vi "Build Update Query.vi"(6 "Where":string, 7 "Schema Name":string, 8 "error in (no error)":errorcluster, 9 "Data":string[](array[string]), 10 "Column Names":string[](array[string]), 11 "Table Name":string) -> (0 "error out":errorcluster, 3 "SQL":string caption="SQL+ (Col[]) VALUES (?[])")   [LabVIEW 2023, in "HardwareAbstractionLayer_LVOOP.lvlib" / "Database.lvclass"]
uses:
  Database.lvclass
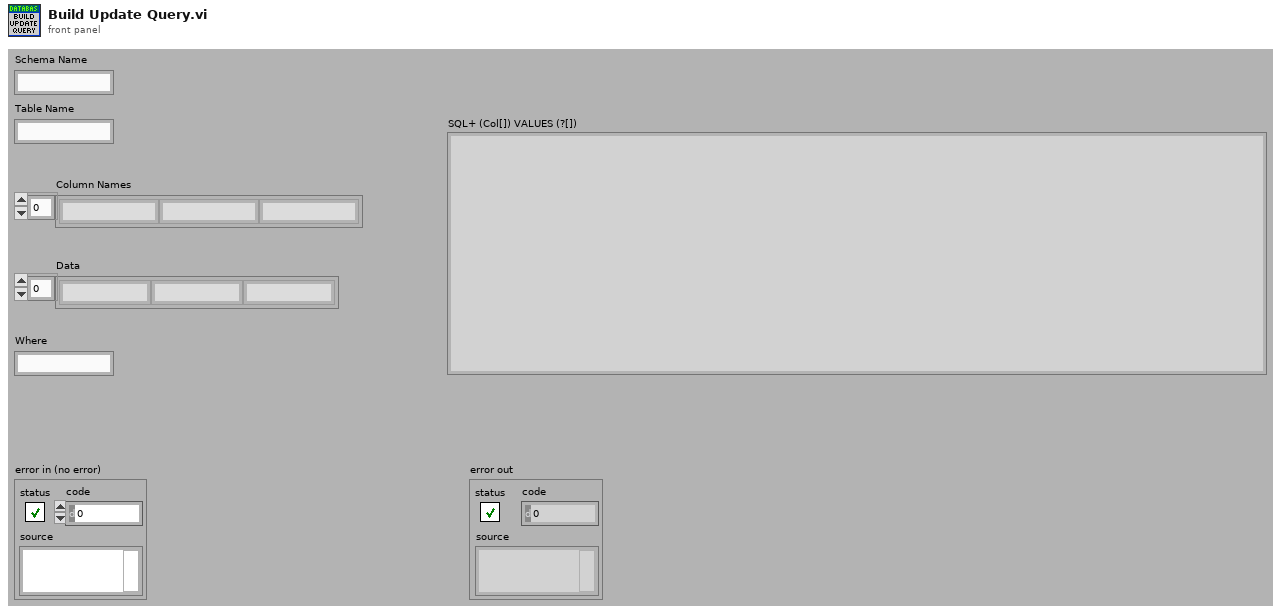
[diagram p1: front panel]
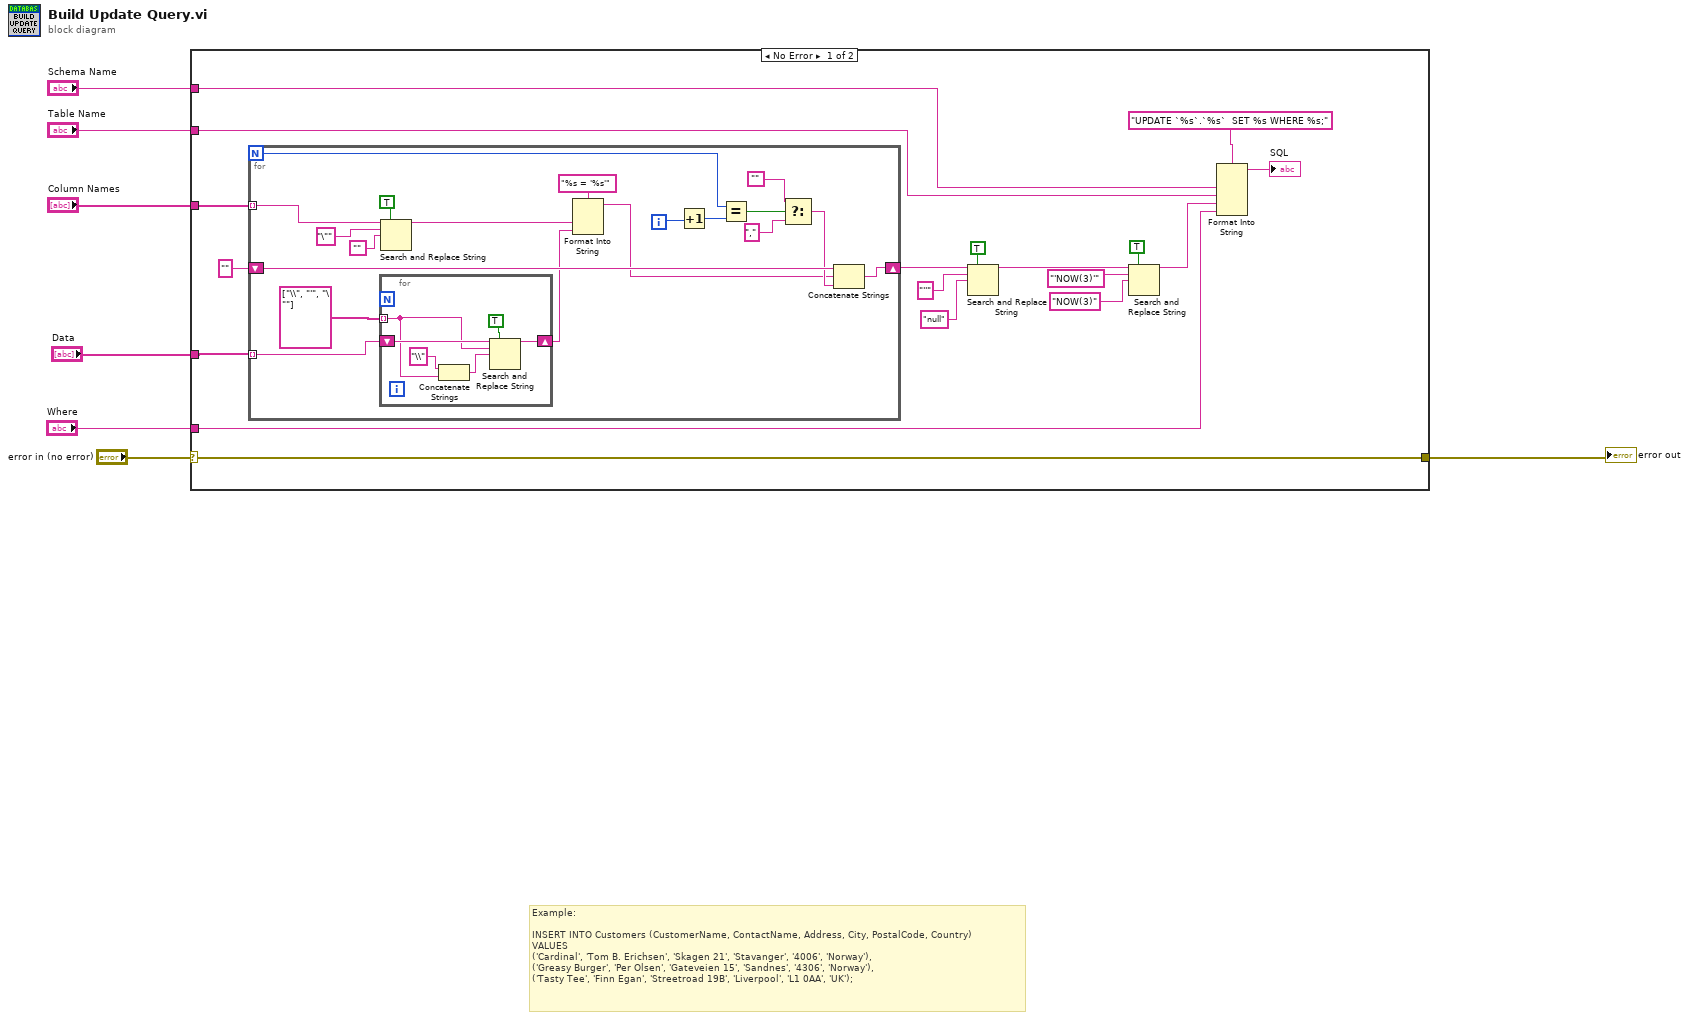
[diagram p0: block diagram]
diagram:
  # "Example:\n\nINSERT INTO Customers (CustomerName, ContactName, Address, City, PostalCode, Country)\nVALUES\n('Cardinal', 'Tom B. Erichsen', 'Skagen 21', 'Stavanger', '4006', 'Norway'),\n('Greasy Burger', 'Per Olsen', 'Gateveien 15', 'Sandnes', '4306', 'Norway'),\n('Tasty Tee', 'Finn Egan', 'Streetroad 19B', 'Liverpool', 'L1 0AA', 'UK');"
  n1 = case shown="No Error" "error in (no error)" {
    selector: "error in (no error)" -> [w25 w51]
    tunnel: [w25 w51] -> w6
    tunnel: "Column Names" -> [w15 _]
    tunnel: "Data" -> [w23 _]
    tunnel: "Table Name" -> [w21 _]
    tunnel: "Where" -> [w14 _]
    tunnel: "Schema Name" -> [w13 _]
    frame No Error {
      n2 = for {
        N -> [w42]
        tunnel: w23 -> [w27] mode=indexing
        shift-right: [w44] -> w19
        shift-left: "" -> [w43]
        tunnel: w15 -> [w32] mode=indexing
        i -> [w41]
        n3 = for {
          tunnel: string[] ["\\", "'", "\""] -> [w45] mode=indexing
          shift-right: [w48] -> w26
          shift-left: w27 -> [w49]
          n4 = Concatenate Strings("\\", w45) -> (w46:string)
          n5 = Search and Replace String(replace all?=TRUE ("replace all? (F)"), input string=w49, search string=w45, replace string=w46) -> (result string=w48:string)  [unwired: 4 in, 3 out]
        }
        n6 = Search and Replace String(replace all?=TRUE ("replace all? (F)"), input string=w32, search string="\"", replace string="") -> (result string=w30:string)  [unwired: 4 in, 3 out]
        n7 = Format Into String(format string="%s = '%s'", w30, w26) -> (resulting string=w29:string)  [unwired: 2 in, 1 out]
        n8 = Increment(x=w41) -> (x+1=w40:i32)
        n9 = Equal?(x=w42, y=w40) -> (x = y?=w39:bool)
        n10 = Select(t="" ("string"), s=w39, f="," ("string")) -> (s? t:f=w37:string)
        n11 = Concatenate Strings(w43, w29, w37) -> (w44:string)
      }
      n12 = Search and Replace String(replace all?=TRUE ("replace all? (F)"), input string=w19, search string="''", replace string="null") -> (result string=w9:string)  [unwired: 4 in, 3 out]
      n13 = Search and Replace String(replace all?=TRUE ("replace all? (F)"), input string=w9, search string="'NOW(3)'", replace string="NOW(3)") -> (result string=w8:string)  [unwired: 4 in, 3 out]
      n14 = Format Into String(format string="UPDATE `%s`.`%s`  SET %s WHERE %s;", w13, w21, w8, w14) -> (resulting string=→"SQL":string)  [unwired: 2 in, 1 out]
    }
    frame Error {
    }
  }
  "error out" <- w6
